vi "Vacuum_tester_interface.vi"() -> ()   [LabVIEW 2017]
uses:
  Type_Defs/TvacStatus.ctl
  <vilib>/httpClient/ClientHandle.ctl
  <vilib>/Utility/error.llb/DialogType.ctl
  msg7171_linux.llb/send single message.vi
  msg7171_linux.llb/send multiple messages.vi
  <vilib>/httpClient/LabVIEWHTTPClient.lvlib
panel:
  out "Cmd Result":string
  in  "Log?":u8(ring) items=["Linear", "Log"]
  in  "Minutes to Display":dbl=5.0
  out "Presure Guages":T1(graph)
  out "Current Vacuum State":string
  in  "Regen":bool
  in  "Vacuum Wanted":bool
  out "TvacStatus":T2
  out "getTvacStatus json":string
  out "getVacuumState json":string
  in  "exit":bool
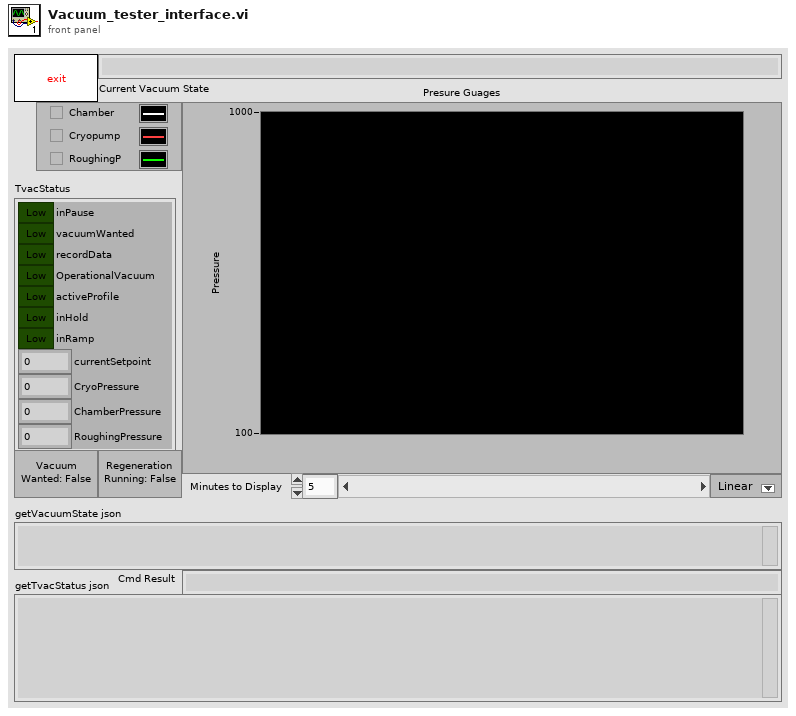
[diagram p1: front panel]
types:
  T1 = cluster{"ChamberPressure":dbl, "CryoPressure":dbl, "RoughingPressure":dbl}
  T2 = typedef "TvacStatus.ctl" = cluster{"inPause":bool, "vacuumWanted":bool, "recordData":bool, "OperationalVacuum":bool, "activeProfile":bool, "inHold":bool, "inRamp":bool, "currentSetpoint":i32, "CryoPressure":dbl, "ChamberPressure":dbl, "RoughingPressure":dbl}
  T3 = typedef "LabVIEWHTTPClient.lvlib/ClientHandle.ctl" = refnum<k1>
  T4 = cluster{"go":bool, "Http session":T3, "URL prefex":string}
  T5 = typedef "DialogType.ctl" = u16
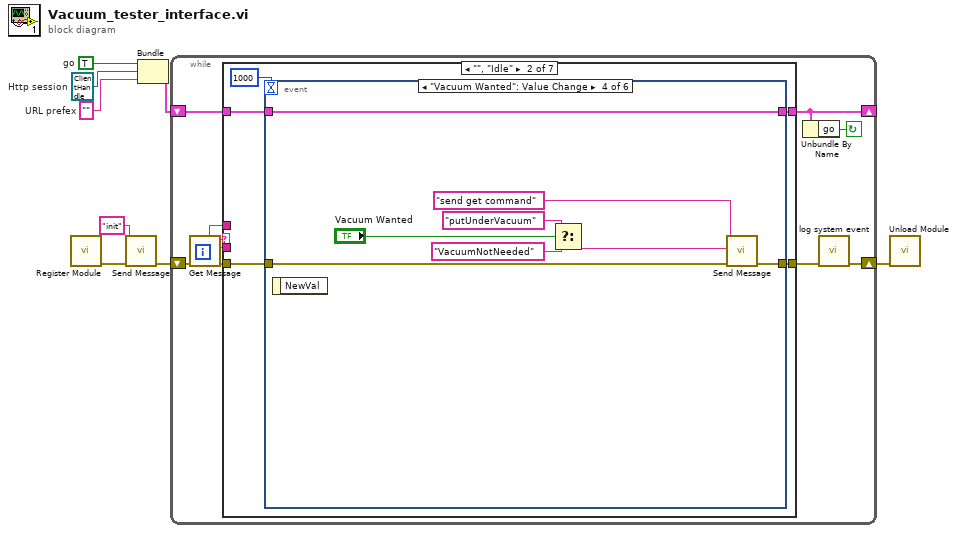
[diagram p0: block diagram]
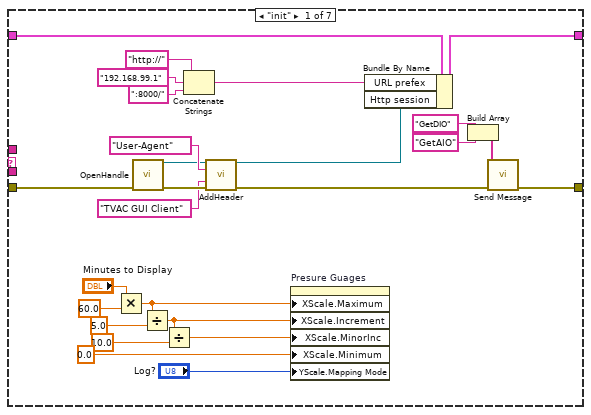
[diagram p2: hidden frame]
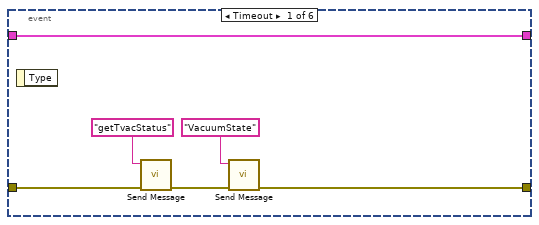
[diagram p3: hidden frame]
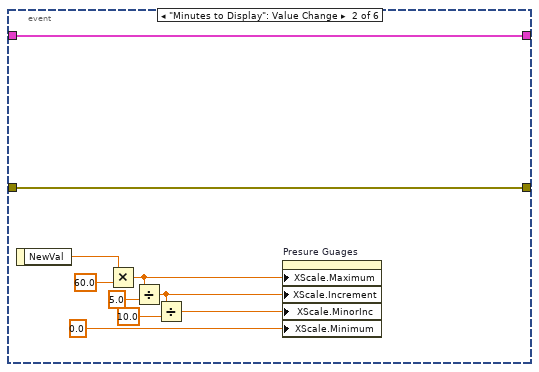
[diagram p4: hidden frame]
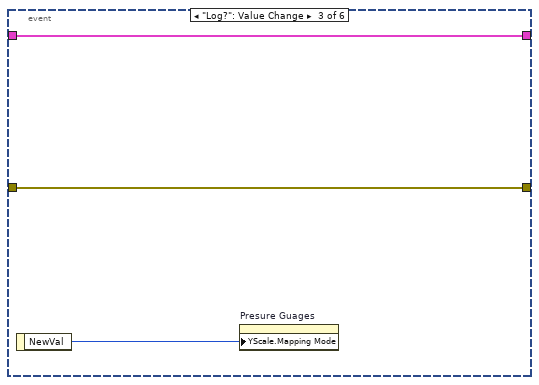
[diagram p5: hidden frame]
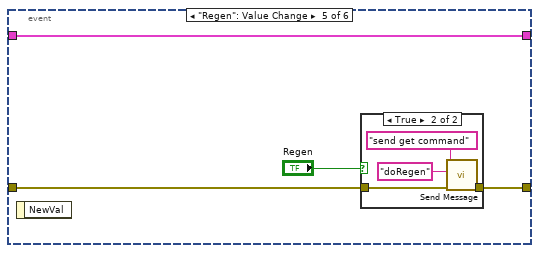
[diagram p6: hidden frame]
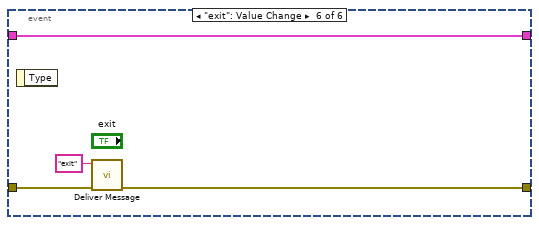
[diagram p8: hidden frame]
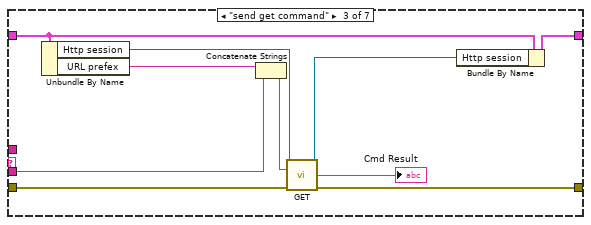
[diagram p9: hidden frame]
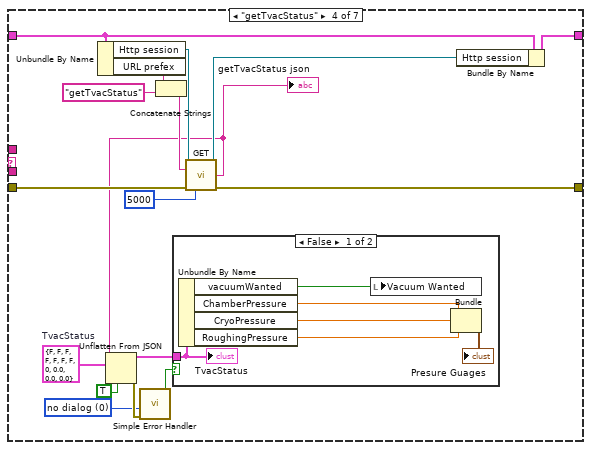
[diagram p10: hidden frame]
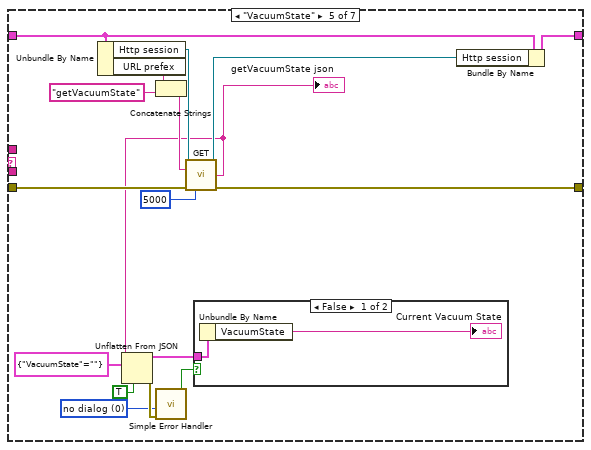
[diagram p12: hidden frame]
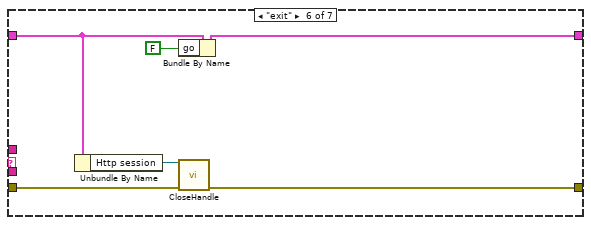
[diagram p14: hidden frame]
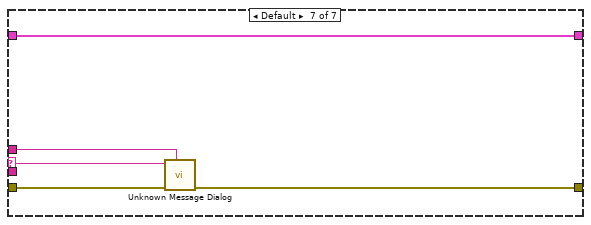
[diagram p15: hidden frame]
diagram:
  w4 = ""  # URL prefex
  w5 = T3 refnum  # Http session
  w6 = TRUE  # go
  n1 = call "Register Module.vi"() -> ("error out"=w2:errorcluster)  [unwired: 10 in, 1 out]
  n2 = call-poly "Send Message.vi"("error in (no error)"=w2, "event"="init") -> ("error out"=w1:errorcluster)  [unwired: 9 in]
  n3 = Bundle("go"=w6, "Http session"=w5, "URL prefex"=w4) -> (w8:T4)  [unwired: 1 in]
  n4 = while {
    shift-left: w8 -> [w15]
    shift-right: [w12] -> _
    shift-right: [w10] -> w7
    shift-left: w1 -> [w18]
    stop <- w11 continue-if-true
    n5 = call "Get Message.vi"("error in (no error)"=w18) -> ("error out"=w16:errorcluster, "event buffer"=w17:string, "event"=w14:string, "source"=w13:string)  [unwired: 7 in]
    n6 = case shown="\"\", \"Idle\"" w14 {
      selector: w14 -> [_ _ _ _ _ _ w150]
      tunnel: [w35 w46 w95 w109 w132 w147 w152] -> w12
      tunnel: w15 -> [w44 w45 w94 w108 w131 w142 w152]
      tunnel: w17 -> [_ _ w90 _ _ _ _]
      tunnel: w16 -> [w39 w47 w93 w111 w134 w145 w151]
      tunnel: w13 -> [_ _ _ _ _ _ w149]
      tunnel: [w31 w49 w92 w110 w133 w144 w148] -> w9
      frame "init" {
        n7 = Multiply(x="Minutes to Display", y=60.0) -> (x*y=w24:dbl)
        n8 = call <vilib>:"OpenHandle.vi"("error in (no error)"=w39) -> ("client handle out"=w40:T3, "error out"=w43:errorcluster)  [unwired: 13 in]
        n9 = Divide(x=w24, y=5.0) -> (x/y=w21:dbl)
        n10 = Divide(x=w21, y=10.0) -> (x/y=w20:dbl)
        n11 = Concatenate Strings("http://" ("url"), "192.168.99.1" ("Address"), ":8000/" ("url")) -> (w34:string)
        n12 = call <vilib>:"AddHeader.vi"("client handle"=w40, "header"="User-Agent", "value"="TVAC GUI Client", "error in (no error)"=w43) -> ("client handle out"=w33:T3, "error out"=w32:errorcluster)  [unwired: 10 in]
        n13 = property on="Presure Guages" class="WFChart (strict)"("XScale.Maximum"=w24, "XScale.Increment"=w21, "XScale.MinorInc"=w20, "XScale.Minimum"=0.0 ("X Scale.Range:Minimum"), "YScale.Mapping Mode"="Log?") -> ()  [unwired: 2 in, 2 out]
        n14 = Bundle By Name(cluster=w44, "URL prefex"=w34, "Http session"=w33) -> (w35:T4)
        n15 = Build Array("GetDIO" ("event"), "GetAIO" ("event")) -> (w29:string[])
        n16 = call-poly "Send Message.vi"("error in (no error)"=w32, "event"=w29) -> ("error out"=w31:errorcluster)  [unwired: 9 in]
      }
      frame "", "Idle" {
        n17 = event shown="[3] \"Vacuum Wanted\": Value Change" {
          selector: _ -> [_ _ _ _ _ _]
          dyn-events: _ -> [_ _ _ _ _ _]
          timeout: 1000 ("milliseconds to wait") -> [_ _ _ _ _ _]
          tunnel: w47 -> [w54 w57 w67 w75 w79 w89]
          tunnel: [w50 w57 w67 w74 w78 w88] -> w49
          tunnel: [w55 w56 w66 w76 w80 w86] -> w46
          tunnel: w45 -> [w55 w56 w66 w76 w80 w86]
          event Timeout {
            n18 = event-data() -> ()  [unwired: 1 in, 1 out]
            n19 = call-poly "Send Message.vi"("error in (no error)"=w54, "event"="getTvacStatus") -> ("error out"=w52:errorcluster)  [unwired: 9 in]
            n20 = call-poly "Send Message.vi"("error in (no error)"=w52, "event"="VacuumState") -> ("error out"=w50:errorcluster)  [unwired: 9 in]
          }
          event "Minutes to Display": Value Change {
            n21 = event-data() -> ("NewVal"=w58:dbl)  [unwired: 1 in]
            n22 = Multiply(x=w58, y=60.0) -> (x*y=w63:dbl)
            n23 = Divide(x=w63, y=5.0) -> (x/y=w60:dbl)
            n24 = Divide(x=w60, y=10.0) -> (x/y=w59:dbl)
            n25 = property on="Presure Guages" class="WFChart (strict)"("XScale.Maximum"=w63, "XScale.Increment"=w60, "XScale.MinorInc"=w59, "XScale.Minimum"=0.0 ("X Scale.Range:Minimum")) -> ()  [unwired: 2 in, 2 out]
          }
          event "Log?": Value Change {
            n26 = event-data() -> ("NewVal"=w68:u8)  [unwired: 1 in]
            n27 = property on="Presure Guages" class="WFChart (strict)"("YScale.Mapping Mode"=w68) -> ()  [unwired: 2 in, 2 out]
          }
          event "Vacuum Wanted": Value Change {
            n28 = event-data() -> ()  [unwired: 1 in, 1 out]
            n29 = Select(t="putUnderVacuum" ("url"), s="Vacuum Wanted", f="VacuumNotNeeded" ("url")) -> (s? t:f=w71:string)
            n30 = call-poly "Send Message.vi"("error in (no error)"=w75, "event buffer"=w71, "event"="send get command") -> ("error out"=w74:errorcluster)  [unwired: 8 in]
          }
          event "Regen": Value Change {
            n31 = event-data() -> ()  [unwired: 1 in, 1 out]
            n32 = case shown="True" "Regen" {
              tunnel: w79 -> [w81 w85]
              tunnel: [w81 w84] -> w78
              frame False {
              }
              frame True {
                n33 = call-poly "Send Message.vi"("error in (no error)"=w85, "event buffer"="doRegen" ("url"), "event"="send get command") -> ("error out"=w84:errorcluster)  [unwired: 8 in]
              }
            }
          }
          event "exit": Value Change {
            n34 = event-data() -> ()  [unwired: 1 in, 1 out]
            n35 = call "Deliver Message.vi"("error in (no error)"=w89, "event"="exit") -> ("error out"=w88:errorcluster)  [unwired: 9 in]
          }
        }
      }
      frame "send get command" {
        n36 = Unbundle By Name(w94) -> ("Http session"=w98:T3, "URL prefex"=w96:string)
        n37 = Concatenate Strings(w96, w90) -> (w97:string)
        n38 = call <vilib>:"GET.vi"("client handle"=w98, "url"=w97, "error in (no error)"=w93) -> ("client handle out"=w99:T3, "body"=→"Cmd Result":string, "error out"=w92:errorcluster)  [unwired: 9 in, 1 out]
        n39 = Bundle By Name(cluster=w94, "Http session"=w99) -> (w95:T4)
      }
      frame "getTvacStatus" {
        w103 = T5 0 items=["no dialog", "OK message", "continue or stop message", "OK message + warnings", "continue/stop + warnings"] ("type of dialog (OK msg:1)")
        w106 = T2 {"inPause"=FALSE, "vacuumWanted"=FALSE, "recordData"=FALSE, "OperationalVacuum"=FALSE, "activeProfile"=FALSE, "inHold"=FALSE, "inRamp"=FALSE, "currentSetpoint"=0, "CryoPressure"=0.0, "ChamberPressure"=0.0, "RoughingPressure"=0.0}  # TvacStatus
        n40 = Unbundle By Name(w108) -> ("Http session"=w115:T3, "URL prefex"=w113:string)
        n41 = Concatenate Strings(w113, "getTvacStatus" ("url")) -> (w114:string)
        n42 = call <vilib>:"GET.vi"("client handle"=w115, "url"=w114, "error in (no error)"=w111, "timeout (10000)"=5000) -> ("client handle out"=w116:T3, "body"=w102:string, "error out"=w110:errorcluster)  [unwired: 8 in, 1 out]
        "getTvacStatus json" <- w102
        n43 = Unflatten From JSON(JSON string=w102, type and defaults=w106, default null elements? (F)=TRUE) -> (value=w105:T2, error out=w104:errorcluster)  [unwired: 4 in]
        n44 = call <vilib>:"Simple Error Handler.vi"("type of dialog (OK msg:1)"=w103, "error in (no error)"=w104) -> ("error?"=w101:bool)  [unwired: 3 in, 4 out]
        n45 = case shown="False" w101 {
          tunnel: w105 -> [w121 _]
          frame False {
            n46 = Unbundle By Name(w121) -> ("vacuumWanted"=w122:bool, "ChamberPressure"=w119:dbl, "CryoPressure"=w118:dbl, "RoughingPressure"=w117:dbl)
            n47 = local write "Vacuum Wanted"(w122) -> ()
            n48 = Bundle("ChamberPressure"=w119, "CryoPressure"=w118, "RoughingPressure"=w117) -> (→"Presure Guages":T1)  [unwired: 1 in]
            "TvacStatus" <- w121
          }
          frame True {
          }
        }
        n49 = Bundle By Name(cluster=w108, "Http session"=w116) -> (w109:T4)
      }
      frame "VacuumState" {
        w127 = T5 0 items=["no dialog", "OK message", "continue or stop message", "OK message + warnings", "continue/stop + warnings"] ("type of dialog (OK msg:1)")
        n50 = Unbundle By Name(w131) -> ("Http session"=w138:T3, "URL prefex"=w136:string)
        n51 = Concatenate Strings(w136, "getVacuumState" ("url")) -> (w137:string)
        n52 = call <vilib>:"GET.vi"("client handle"=w138, "url"=w137, "error in (no error)"=w134, "timeout (10000)"=5000) -> ("client handle out"=w139:T3, "body"=w124:string, "error out"=w133:errorcluster)  [unwired: 8 in, 1 out]
        "getVacuumState json" <- w124
        n53 = Unflatten From JSON(JSON string=w124, type and defaults=cluster{"VacuumState":string} {"VacuumState"=""}, default null elements? (F)=TRUE) -> (value=w129:cluster{"VacuumState":string}, error out=w128:errorcluster)  [unwired: 4 in]
        n54 = call <vilib>:"Simple Error Handler.vi"("type of dialog (OK msg:1)"=w127, "error in (no error)"=w128) -> ("error?"=w126:bool)  [unwired: 3 in, 4 out]
        n55 = case shown="False" w126 {
          tunnel: w129 -> [w141 _]
          frame False {
            n56 = Unbundle By Name(w141) -> ("VacuumState"=→"Current Vacuum State":string)
          }
          frame True {
          }
        }
        n57 = Bundle By Name(cluster=w131, "Http session"=w139) -> (w132:T4)
      }
      frame "exit" {
        n58 = Unbundle By Name(w142) -> ("Http session"=w143:T3)
        n59 = Bundle By Name(cluster=w142, "go"=FALSE ("Bundle Element")) -> (w147:T4)
        n60 = call <vilib>:"CloseHandle.vi"("client handle"=w143, "error in (no error)"=w145) -> ("error out"=w144:errorcluster)  [unwired: 13 in]
      }
      frame Default {
        n61 = call "Unknown Message Dialog.vi"("source"=w149, "error in (no error)"=w151, "event name"=w150) -> ("error out"=w148:errorcluster)  [unwired: 8 in]
      }
    }
    n62 = Unbundle By Name(w12) -> ("go"=w11:bool)
    n63 = call "log system event.vi"("error in (no error)"=w9) -> ("error out"=w10:errorcluster)  [unwired: 9 in, 1 out]
  }
  n64 = call "Unload Module.vi"("error in (no error)"=w7) -> ()  [unwired: 10 in, 1 out]
